vi "TcA01-005_ObjectCreationAndDestructionWithGenericConstructor.vi"(1 "Input buffer":T3="1", 3 "Invocation info":T2, 5 "error in (no error)":errorcluster, 6 "Add log to result?":bool) -> (16 "Test Data":T1 {"Numeric Measurement" format="%.2f"}, 19 "error out":errorcluster)   [LabVIEW 2020]
doc: "Test case template."
uses:
  Shared/Support_InputBuffer.ctl
  Shared/Support_InvocationInfo.ctl
  Shared/Support_TestData.ctl
  TestClasses/G#SubSubClass1_class/G#SubSubClass1.lvclass
  C:/Projects/GsharpGIT/Verification/TestCases/TestClasses/G#BaseClass1_class/G#BaseClass1.lvclass
  TestClasses/G#SubClass1_class/G#SubClass1.lvclass
  TestClasses/G#BaseClass1_class/G#BaseClass1.lvclass
  <vilib>/addons/_AddQ/G#Object/G#Object.lvclass
panel:
  in  "Test name":string="TcA01-005 Object creation and destruction with generic constructor"
  out "Test result":bool
  out "Result":string
  # "Verify that multiple objects of a base class can\nbe created and destructed multiple times."
  # "Sub test case"
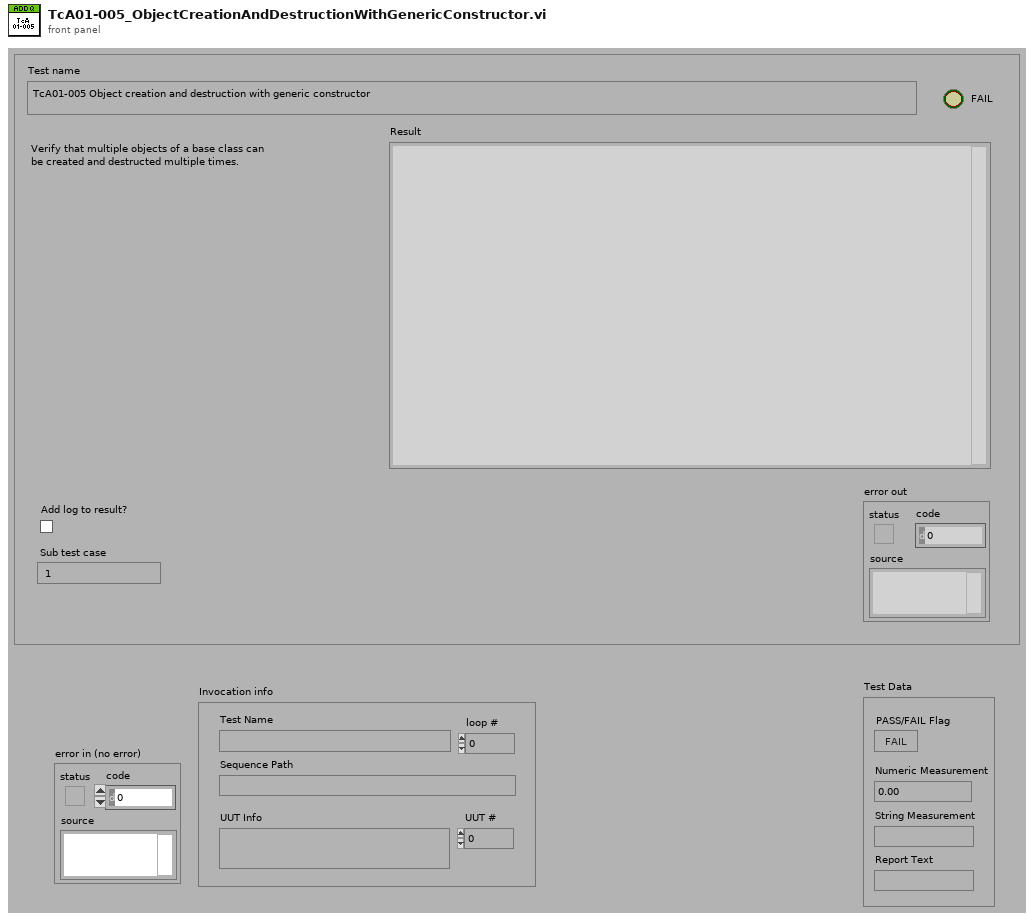
[diagram p1: front panel]
types:
  T1 = typedef "Support_TestData.ctl" = cluster{"PASS/FAIL Flag":bool, "Numeric Measurement":dbl, "String Measurement":string, "Report Text":string}
  T2 = typedef "Support_InvocationInfo.ctl" = cluster{"UUT #":i32, "loop #":i32, "UUT Info":string, "Test Name":string, "Sequence Path":path}
  T3 = typedef "Support_InputBuffer.ctl" = string
  T4 = typedef "Support_ResultType.ctl" = cluster{"Pass":bool, "Comment":string, "MeasurementValue":dbl}
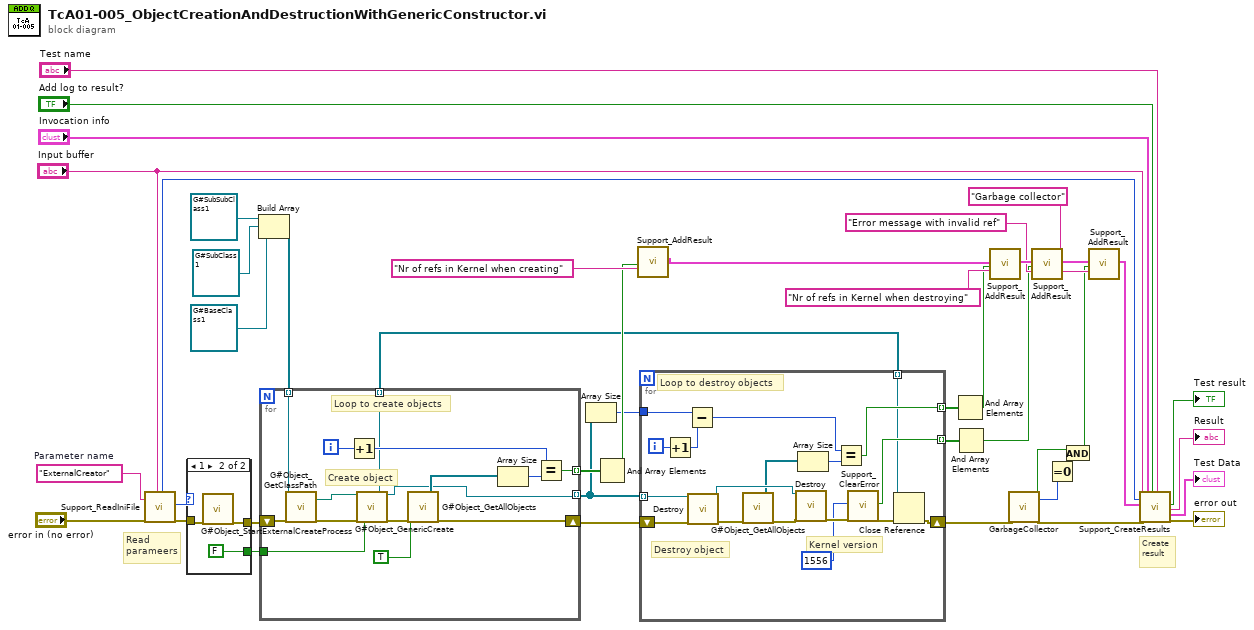
[diagram p0: block diagram]
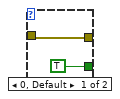
[diagram p2: hidden frame]
diagram:
  w37 = "ExternalCreator"  # Parameter name
  # "Read\nparameers"
  # "Create\nresult"
  n1 = call "Support_ReadIniFile.vi"("Parameter name"=w37, "error in (no error)"="error in (no error)", "Sub test case"="Input buffer") -> ("Timer start"=w26:u32, "Parameter1 as I32"=w4:i32, "error out"=w5:errorcluster)  [unwired: 9 in, 5 out]
  n2 = case shown="1" w4 {
    tunnel: w5 -> [w45 w48]
    tunnel: [w45 w47] -> w3
    tunnel: [TRUE FALSE] -> w1
    frame 0, Default {
    }
    frame 1 {
      n3 = call <vilib>:"G#Object_StartExternalCreateProcess.vi"("error in (no error)"=w48) -> ("error out"=w47:errorcluster)  [unwired: 18 in]
    }
  }
  n4 = Build Array(refnum<class "G#SubSubClass1.lvclass"> refnum ("G#SubSubClass1.lvclass"), refnum<class "G#SubClass1.lvclass"> refnum ("G#SubClass1.lvclass"), refnum<class "G#BaseClass1.lvclass"> refnum ("G#BaseClass1.lvclass")) -> (w8:refnum<class "G#BaseClass1.lvclass">[])
  n5 = for {
    shift-right: [w56] -> w32
    shift-left: w3 -> [w54]
    tunnel: [w55] -> w6 mode=indexing
    tunnel: [w60] -> w35 mode=indexing
    tunnel: w8 -> [w52] mode=indexing
    tunnel: [w50] -> w2 mode=indexing
    tunnel: w1 -> [w49]
    i -> [w63]
    # "Create object"
    # "Loop to create objects"
    n6 = call-dynamic "G#Object_GetClassPath.vi"("reference in"=w52, "error in (no error)"=w54) -> ("class path"=w51:path, "error out"=w53:errorcluster)  [unwired: 15 in, 1 out]
    n7 = Increment(x=w63) -> (x+1=w61:i32)
    n8 = call <vilib>:"G#Object_GenericCreate.vi"("class path"=w51, "error in (no error)"=w53, "respond to create event? (T)"=w49) -> ("constructor VI ref"=w50:refnum<vi>, "reference out"=w55:refnum<class "G#Object.lvclass">, "error out"=w59:errorcluster)  [unwired: 14 in]
    n9 = call <vilib>:"G#Object_GetAllObjects.vi"("only refs (F)"=TRUE ("only refs"), "error in (no error)"=w59) -> ("all refs"=w58:refnum<class "G#Object.lvclass">[], "error out"=w56:errorcluster)  [unwired: 14 in, 2 out]
    n10 = Array Size(array=w58) -> (size(s)=w62:i32)
    n11 = Equal?(x=w61, y=w62) -> (x = y?=w60:bool)
  }
  n12 = Array Size(array=w6) -> (size(s)=w7:i32)
  n13 = And Array Elements(Boolean array=w35) -> (logical AND=w33:bool)
  n14 = call "Support_AddResult.vi"("Pass"=w33, "Comment"="Nr of refs in Kernel when creating") -> ("Results out"=w21:T4[])  [unwired: 17 in]
  n15 = for {
    shift-right: [w66] -> w20
    shift-left: w32 -> [w79]
    tunnel: [w80] -> w31 mode=indexing
    tunnel: w6 -> [w75] mode=indexing
    tunnel: w7 -> [w78]
    tunnel: [w71] -> w25 mode=indexing
    tunnel: w2 -> [w64] mode=indexing
    i -> [w81]
    # "Destroy object"
    # "Loop to destroy objects"
    # "Kernel version"
    n16 = Increment(x=w81) -> (x+1=w77:i32)
    n17 = Subtract(x=w78, y=w77) -> (x-y=w76:i32)
    n18 = call-dynamic "Destroy.vi"("reference in"=w75, "error in (no error)"=w79) -> ("reference out"=w70:refnum<class "G#Object.lvclass">, "error out"=w67:errorcluster)  [unwired: 16 in]
    n19 = call <vilib>:"G#Object_GetAllObjects.vi"("error in (no error)"=w67) -> ("all refs"=w68:refnum<class "G#Object.lvclass">[], "error out"=w69:errorcluster)  [unwired: 15 in, 2 out]
    n20 = call-dynamic "Destroy.vi"("reference in"=w70, "error in (no error)"=w69) -> ("error out"=w73:errorcluster)  [unwired: 16 in, 1 out]
    n21 = Array Size(array=w68) -> (size(s)=w74:i32)
    n22 = Equal?(x=w76, y=w74) -> (x = y?=w80:bool)
    n23 = call "Support_ClearError.vi"("code"=1556, "error in (no error)"=w73) -> ("Cleared?"=w71:bool, "error out"=w65:errorcluster)  [unwired: 16 in]
    n24 = Close Reference(reference=w64, error in (no error)=w65) -> (error out=w66:errorcluster)
  }
  n25 = And Array Elements(Boolean array=w31) -> (logical AND=w29:bool)
  n26 = And Array Elements(Boolean array=w25) -> (logical AND=w22:bool)
  n27 = call "Support_AddResult.vi"("Results in"=w21, "Pass"=w29, "Comment"="Nr of refs in Kernel when destroying") -> ("Results out"=w24:T4[])  [unwired: 16 in]
  n28 = call <vilib>:"GarbageCollector.vi"("error in (no error)"=w20) -> ("OK"=w15:bool, "# of objects killed"=w13:i32, "error out"=w19:errorcluster)  [unwired: 16 in]
  n29 = call "Support_AddResult.vi"("Results in"=w24, "Pass"=w22, "Comment"="Error message with invalid ref") -> ("Results out"=w18:T4[])  [unwired: 16 in]
  n30 = Equal To 0?(x=w13) -> (x = 0?=w14:bool)
  n31 = And(x=w15, y=w14) -> (x .and. y?=w12:bool)
  n32 = call "Support_AddResult.vi"("Results in"=w18, "Pass"=w12, "Comment"="Garbage collector") -> ("Results out"=w17:T4[])  [unwired: 16 in]
  n33 = call "Support_CreateResults.vi"("Sub test case"="Input buffer", "Timer start"=w26, "Results"=w17, "error in (no error)"=w19, "Invocation info"="Invocation info", "Add log to result?"="Add log to result?", "Test name"="Test name") -> ("Pass/fail flag"=→"Test result":bool, "Result"=→"Result":string, "Test Data"=→"Test Data":T1, "error out"=→"error out":errorcluster)  [unwired: 9 in]
